vi "Read.vi"(4 "TypeMap in":refnum<class "TypeMap.lvclass">, 6 "commandTimeout":i32, 8 "error in (no error)":errorcluster, 9 "Where":string, 10 "object in":refnum<class>, 11 "SqlMapper in":refnum<class "SqlMapper.lvclass">) -> (0 "error out":errorcluster, 1 "NotFound":bool, 2 "Value":refnum<class>, 3 "SqlMapper out":refnum<class "SqlMapper.lvclass">)   [LabVIEW 2020, in "ORM.lvlib" / "TypeMap.lvclass"]
uses:
  TypeMap.lvclass
  SqlMapper/SqlMapper.lvclass
  Read Table Name.vi
  TypeMap.lvclass/TypeMap.ctl
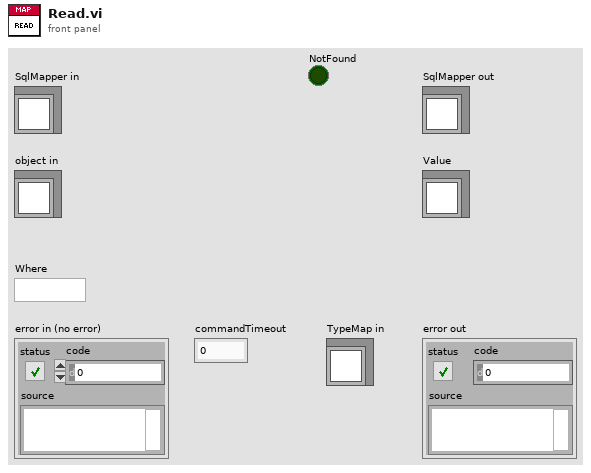
[diagram p1: front panel]
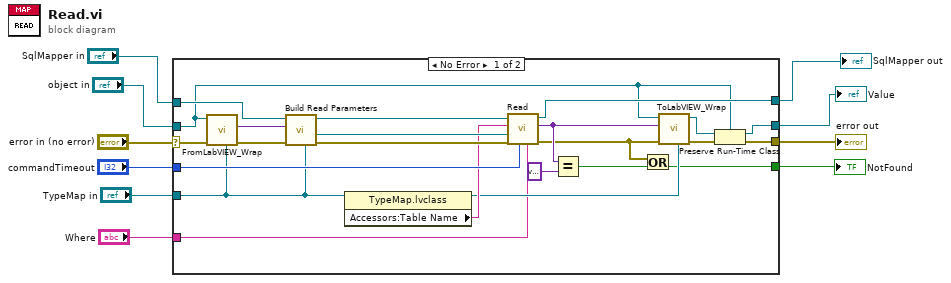
[diagram p0: block diagram]
diagram:
  n1 = case shown="No Error" "error in (no error)" {
    selector: "error in (no error)" -> [w33 w34]
    tunnel: "object in" -> [w11 w35]
    tunnel: "SqlMapper in" -> [w16 w36]
    tunnel: [w14 w34] -> w7
    tunnel: [w15 w36] -> w6
    tunnel: [w12 w35] -> w5
    tunnel: "commandTimeout" -> [w30 _]
    tunnel: "TypeMap in" -> [w26 _]
    tunnel: "Where" -> [w23 _]
    tunnel: [w19 _] -> w1
    frame No Error {
      n2 = call "FromLabVIEW_Wrap.vi"("TypeMap in"=w26, "error in (no error)"=w33, "object in"=w11) -> ("error out"=w31:errorcluster, "DbRow"=w17:variant)  [unwired: 7 in]
      n3 = call-dynamic "Build Read Parameters.vi"("TypeMap in"=w26, "error in (no error)"=w31, "object"=w17, "SqlMapper in"=w16) -> ("error out"=w29:errorcluster, "DynamicParameters out"=w27:refnum<class "DynamicParameters.lvclass">, "SqlMapper out"=w28:refnum<class "SqlMapper.lvclass">)  [unwired: 5 in]
      n4 = property class="TypeMap.lvclass"(reference=w26) -> (reference out=w24:refnum<class "TypeMap.lvclass">, "Accessors:Table Name"=w25:string)  [unwired: 1 in, 1 out]
      n5 = call "Read.vi"("Where"=w23, "commandTimeout"=w30, "error in (no error)"=w29, "DynamicParameters"=w27, "TableName"=w25, "SqlMapper in"=w28) -> ("error out"=w18:errorcluster, "Value"=w22:variant, "SqlMapper out"=w15:refnum<class "SqlMapper.lvclass">)  [unwired: 3 in]
      n6 = Equal?(x=w22, y=variant) -> (x = y?=w20:bool)
      n7 = Or(x=w18, y=w20) -> (x .or. y?=w19:bool)
      n8 = call "ToLabVIEW_Wrap.vi"("TypeMap in"=w24, "error in (no error)"=w18, "DbRow"=w22, "TargetObject In"=w11) -> ("error out"=w32:errorcluster, "Object Out"=w13:refnum<class>)  [unwired: 6 in]
      n9 = Preserve Run-Time Class(object in=w13, error in=w32, 2:w11) -> (object out=w12:refnum<class>, error out=w14:errorcluster)
    }
    frame Error {
    }
  }
  "Value" <- w5
  "error out" <- w7
  "SqlMapper out" <- w6
  "NotFound" <- w1
